vi "Core.vi"(8 "error in (no error)":errorcluster, 11 "HSMS Class in":refnum<class "HSMS Class.lvclass">) -> (0 "error out":errorcluster, 3 "HSMS Class out":refnum<class "HSMS Class.lvclass">)   [LabVIEW 2020, in "SECS Communication.lvlib" / "HSMS Class.lvclass"]
uses:
  HSMS Class.lvclass
  HSMS State.ctl
  HSMS Class.lvclass/HSMS Class.ctl
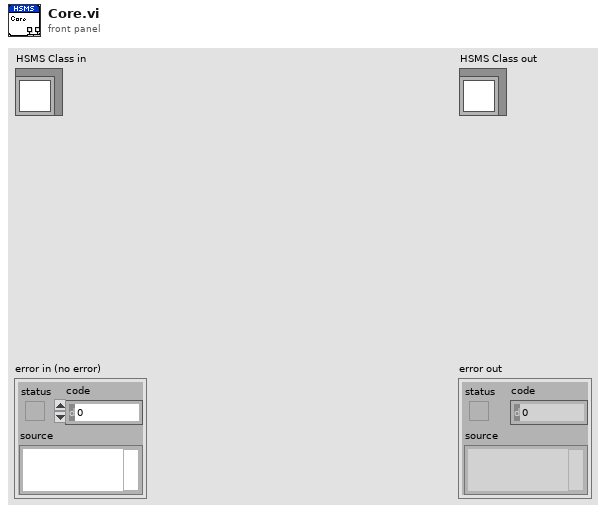
[diagram p1: front panel]
types:
  T1 = typedef "SECS Communication.lvlib/HSMS Class.lvclass/HSMS State.ctl" = enum16{"[TCP/IP]Not Connect", "[HSMS]Not Selected", "[HSMS]Selected", "Stop"}
  T2 = typedef "SECS Communication.lvlib/HSMS Class.lvclass/Notifier Data.ctl" = cluster{"Notifier Type":T3, "Data":variant, "Time":timestamp}
  T3 = typedef "SECS Communication.lvlib/HSMS Class.lvclass/Notifier Type.ctl" = enum16{"TCPIP Connect", "TCPIP Disconnect", "Receive Message", "Send Message", "T3 Timeout", "T6 Timeout", "T7 Timeout", "Error", "Stop"}
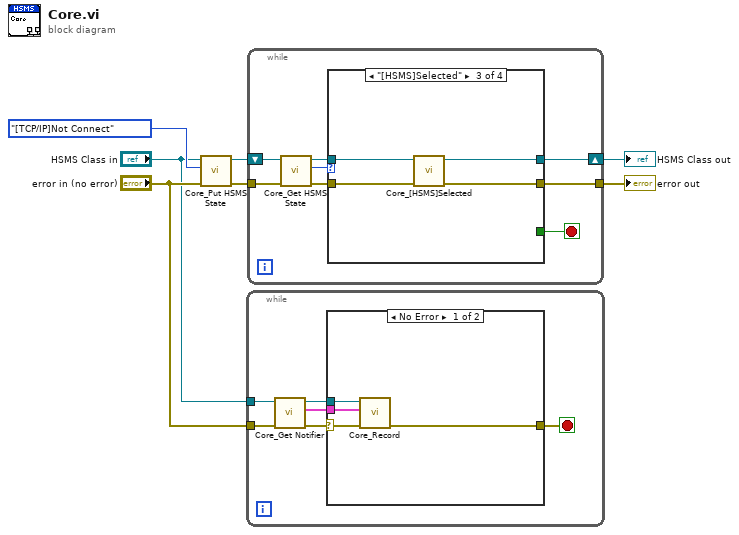
[diagram p0: block diagram]
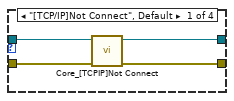
[diagram p3: hidden frame]
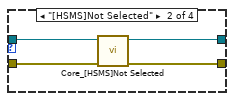
[diagram p4: hidden frame]
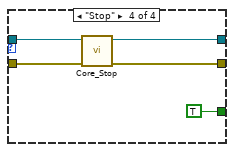
[diagram p5: hidden frame]
diagram:
  n1 = call "Core_Put HSMS State.vi"("error in (no error)"="error in (no error)", "HSMS State"=HSMS_State."[TCP/IP]Not Connect", "HSMS Class in"="HSMS Class in") -> ("error out"=w5:errorcluster, "HSMS Class out"=w3:refnum<class "HSMS Class.lvclass">)  [unwired: 7 in]
  n2 = while {
    tunnel: "error in (no error)" -> [w13]
    tunnel: "HSMS Class in" -> [w12]
    stop <- w8 stop-if-true
    n3 = call "Core_Get Notifier.vi"("error in (no error)"=w13, "HSMS Class in"=w12) -> ("error out"=w11:errorcluster, "Notifier Data"=w9:T2, "HSMS Class out"=w10:refnum<class "HSMS Class.lvclass">)  [unwired: 7 in]
    n4 = case shown="No Error" w11 {
      selector: w11 -> [w17 w18]
      tunnel: w10 -> [w15 _]
      tunnel: w9 -> [w16 _]
      tunnel: [w14 w18] -> w8
      frame No Error {
        n5 = call "Core_Record.vi"("error in (no error)"=w17, "Notifier Data"=w16, "HSMS Class in"=w15) -> ("error out"=w14:errorcluster)  [unwired: 7 in, 1 out]
      }
      frame Error {
      }
    }
  }
  n6 = while {
    tunnel: w5 -> [w26]
    tunnel: [w21] -> w6
    shift-right: [w20] -> w7
    shift-left: w3 -> [w25]
    stop <- w19 stop-if-true
    n7 = call "Core_Get HSMS State.vi"("error in (no error)"=w26, "HSMS Class in"=w25) -> ("error out"=w24:errorcluster, "HSMS State"=w23:T1, "HSMS Class out"=w22:refnum<class "HSMS Class.lvclass">)  [unwired: 7 in]
    n8 = case shown="\"[HSMS]Selected\"" w23 {
      tunnel: w24 -> [w30 w34 w38 w42]
      tunnel: w22 -> [w29 w33 w37 w41]
      tunnel: [w28 w31 w35 w39] -> w21
      tunnel: [w27 w32 w36 w40] -> w20
      tunnel: [_ _ _ TRUE] -> w19
      frame "[TCP/IP]Not Connect", Default {
        n9 = call "Core_[TCPIP]Not Connect.vi"("error in (no error)"=w30, "HSMS Class in"=w29) -> ("error out"=w28:errorcluster, "HSMS Class out"=w27:refnum<class "HSMS Class.lvclass">)  [unwired: 8 in]
      }
      frame "[HSMS]Not Selected" {
        n10 = call "Core_[HSMS]Not Selected.vi"("error in (no error)"=w34, "HSMS Class in"=w33) -> ("error out"=w31:errorcluster, "HSMS Class out"=w32:refnum<class "HSMS Class.lvclass">)  [unwired: 8 in]
      }
      frame "[HSMS]Selected" {
        n11 = call "Core_[HSMS]Selected.vi"("error in (no error)"=w38, "HSMS Class in"=w37) -> ("error out"=w35:errorcluster, "HSMS Class out"=w36:refnum<class "HSMS Class.lvclass">)  [unwired: 8 in]
      }
      frame "Stop" {
        n12 = call "Core_Stop.vi"("error in (no error)"=w42, "HSMS Class in"=w41) -> ("error out"=w39:errorcluster, "HSMS Class out"=w40:refnum<class "HSMS Class.lvclass">)  [unwired: 8 in]
      }
    }
  }
  "error out" <- w6
  "HSMS Class out" <- w7
